vi "toTypeTag.vi"(9 "Tags":string[](array[string]), 10 "permission":string, 11 "type":string) -> (3 "typeTags":T1)   [LabVIEW 2013]
uses:
  TypeTags.ctl
  TagPermission.ctl
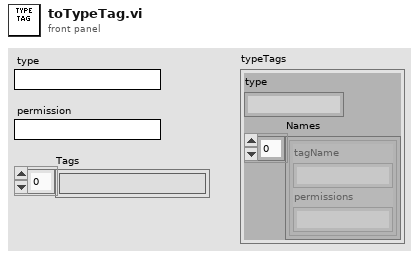
[diagram p1: front panel]
types:
  T1 = typedef "TypeTags.ctl" = cluster{"type":string, "Names":T2[]}
  T2 = typedef "TagPermission.ctl" = cluster{"tagName":string, "permissions":string}
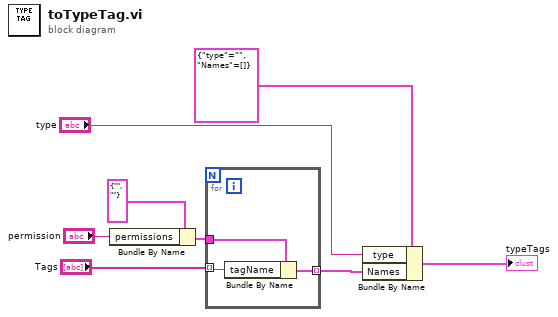
[diagram p0: block diagram]
diagram:
  n1 = Bundle By Name(cluster=T2 {"tagName"="", "permissions"=""} ("TagPermission"), "permissions"="permission") -> (w6:T2)
  n2 = for {
    tunnel: w6 -> [w11]
    tunnel: "Tags" -> [w10] mode=indexing
    tunnel: [w9] -> w2 mode=indexing
    n3 = Bundle By Name(cluster=w11, "tagName"=w10) -> (w9:T2)
  }
  n4 = Bundle By Name(cluster=T1 {"type"="", "Names"=[]} ("typeTags"), "type"="type", "Names"=w2) -> (→"typeTags":T1)
